vi "AddModule.vi"(4 "Python module  name":string, 5 "Python module":string, 6 "error in":errorcluster, 9 "PythonConverter in":refnum<class "PythonBDConverter.lvclass">) -> (0 "error out":errorcluster, 3 "PythonConverter out":refnum<class "PythonBDConverter.lvclass">)   [LabVIEW 2014, in "PythonBDConverter.lvclass"]
uses:
  PythonBDConverter.lvclass
  PythonBDConverter.lvclass/PythonBDConverter.ctl
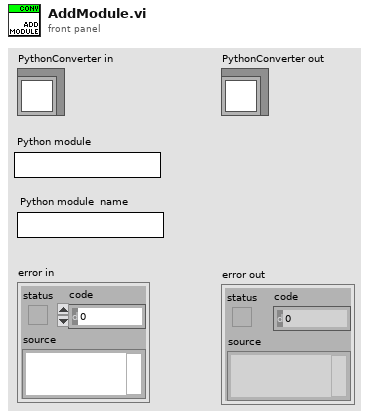
[diagram p1: front panel]
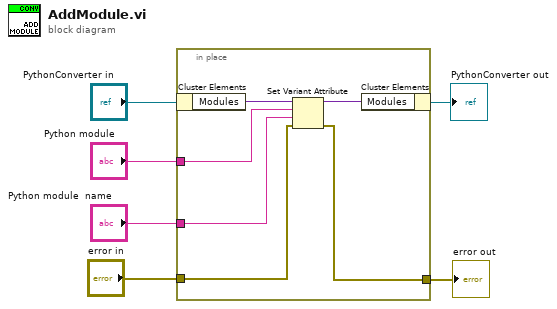
[diagram p0: block diagram]
diagram:
  n1 = in-place {
    in-place-border: "error in" -> [w10]
    in-place-border: [w9] -> w3
    in-place-border: "Python module" -> [w8]
    in-place-border: "Python module  name" -> [w7]
    n2 = in-place-cluster #1("PythonConverter in") -> ("Modules"=w12:variant)
    n3 = Set Variant Attribute(Variant=w12, name=w8, value=w7, error in=w10) -> (Variant out=w11:variant, error out=w9:errorcluster)  [unwired: 1 out]
    n4 = in-place-cluster #1("Modules"=w11) -> (→"PythonConverter out":refnum<class "PythonBDConverter.lvclass">)
  }
  "error out" <- w3
